vi "FdxCmdTxUDPChgSrcPortCvi.vi"(8 "error in":errorcluster, 9 "TxUDPChgSrcPort":cluster{"UdpHandle":u32, "UdpSrc":u32}, 11 "InstrumentHandle":u32) -> (0 "error out":errorcluster, 3 "InstrumentHandle":u32)   [LabVIEW 2020, in "AIM664LV.lvlib"]
doc: "This function is used to change source of a defined UDP queuing port. This function can be\nused if transmitter is running."
uses:
  AIM664LV.lvlib
  AFDX_LibraryAdmin/FdxGlobalDllPath.vi
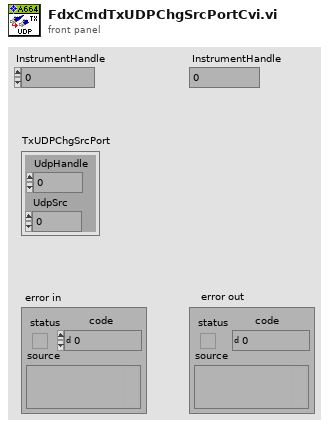
[diagram p1: front panel]
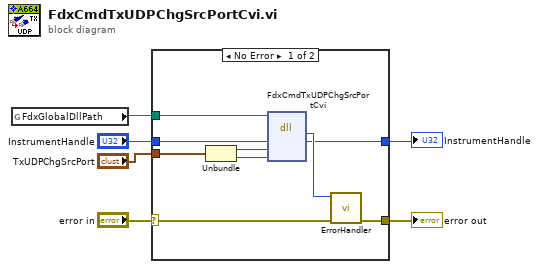
[diagram p0: block diagram]
diagram:
  n1 = global read "FdxGlobalDllPath.vi" "FdxGlobalDllPath"() -> (w4:path)
  n2 = case shown="No Error" "error in" {
    selector: "error in" -> [w14 w17]
    tunnel: [w15 w17] -> w6
    tunnel: w4 -> [w10 _]
    tunnel: [w9 w16] -> w3
    tunnel: "TxUDPChgSrcPort" -> [w8 _]
    tunnel: "InstrumentHandle" -> [w7 w16]
    frame No Error {
      n3 = Unbundle(w8) -> ("UdpHandle"=w12:u32, "UdpSrc"=w11:u32)
      n4 = dll-call lib="aim_fdx.19.dll" fn="FdxCmdTxUDPChgSrcPortCvi"(path in=w10, "InstrumentHandle"=w7, "UdpHandle"=w12, "UdpSrc"=w11) -> ("status"=w13:i32, "InstrumentHandle"=w9:u32)  [unwired: 3 in, 3 out]
      n5 = call "ErrorHandler.vi"("error in"=w14, "AIM Error"=w13) -> ("error out"=w15:errorcluster)  [unwired: 9 in]
    }
    frame Error {
    }
  }
  "error out" <- w6
  "InstrumentHandle" <- w3
